vi "ke37xx Configure Limits.vi"(0 "VISA Resource Name":refnum<visa-resource-name>, 5 "Limit Enabled (False)":bool, 7 "Auto Clear Enabled (False)":bool, 9 "Limit Line (1)":u8=1 min=1 max=2, 11 "error in (no error)":errorcluster, 12 "Lower Limit (NaN: Don't Set)":dbl=nan, 13 "Upper Limit (NaN: Don't Set)":dbl=nan) -> (4 "VISA Resource Name Out":refnum<visa-resource-name>, 15 "error out":errorcluster)   [LabVIEW 2009, in "Keithley 3700 Series.lvlib"]
doc: "This VI allows you to configure the limit testing system for the DMM."
uses:
  <instrlib>/Keithley 3706/Keithley 3700 Series.lvlib
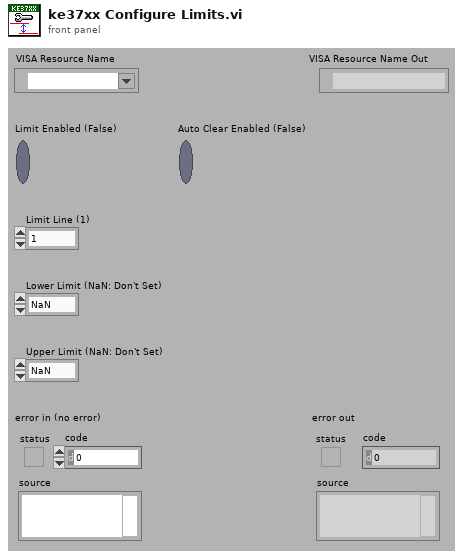
[diagram p1: front panel]
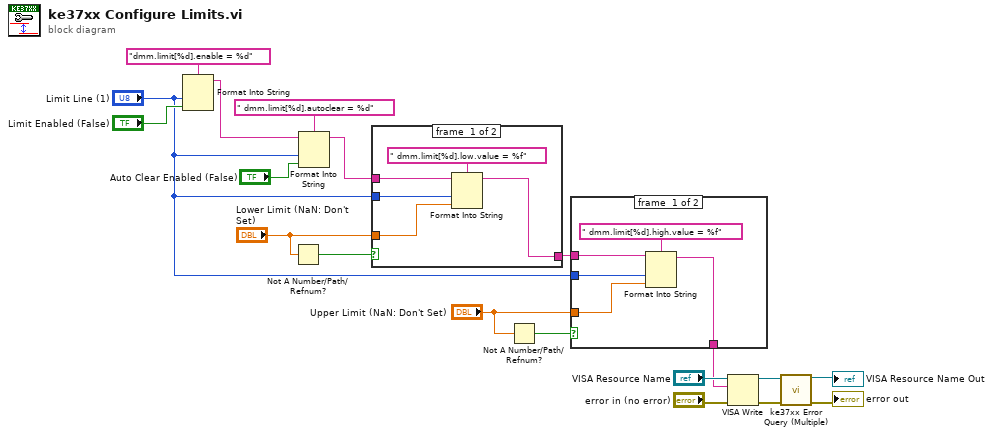
[diagram p0: block diagram]
diagram:
  n1 = Format Into String(format string="dmm.limit[%d].enable = %d", "Limit Line (1)", "Limit Enabled (False)") -> (resulting string=w12:string)  [unwired: 2 in, 1 out]
  n2 = Not A Number/Path/Refnum?(number/path/refnum="Lower Limit (NaN: Don't Set)") -> (NaN/Path/Refnum?=w4:bool)
  n3 = Format Into String(format string=" dmm.limit[%d].autoclear = %d", initial string=w12, "Limit Line (1)", "Auto Clear Enabled (False)") -> (resulting string=w11:string)  [unwired: 1 in, 1 out]
  n4 = case shown="True" w4 {
    tunnel: w11 -> [w24 w25]
    tunnel: [w23 w25] -> w10
    tunnel: "Limit Line (1)" -> [w21 _]
    tunnel: "Lower Limit (NaN: Don't Set)" -> [w20 _]
    frame #0 {
      n5 = Format Into String(format string=" dmm.limit[%d].low.value = %f", initial string=w24, w21, w20) -> (resulting string=w23:string)  [unwired: 1 in, 1 out]
    }
    frame #1 {
    }
  }
  n6 = Not A Number/Path/Refnum?(number/path/refnum="Upper Limit (NaN: Don't Set)") -> (NaN/Path/Refnum?=w2:bool)
  n7 = case shown="True" w2 {
    tunnel: w10 -> [w30 w31]
    tunnel: [w29 w31] -> w9
    tunnel: "Limit Line (1)" -> [w27 _]
    tunnel: "Upper Limit (NaN: Don't Set)" -> [w26 _]
    frame #0 {
      n8 = Format Into String(format string=" dmm.limit[%d].high.value = %f", initial string=w30, w27, w26) -> (resulting string=w29:string)  [unwired: 1 in, 1 out]
    }
    frame #1 {
    }
  }
  n9 = VISA Write(VISA resource name="VISA Resource Name", write buffer=w9, error in (no error)="error in (no error)") -> (VISA resource name out=w14:refnum<visa-resource-name>, error out=w13:errorcluster)  [unwired: 1 out]
  n10 = call <instrlib>:"ke37xx Error Query (Multiple).vi"("VISA resource name"=w14, "error in (no error)"=w13) -> ("VISA resource name out"=→"VISA Resource Name Out":refnum<visa-resource-name>, "error out"=→"error out":errorcluster)  [unwired: 12 out]
